vi "Read Resistance Setpoint.vi"   [LabVIEW 2023, in "Resistance Control.lvclass"]
uses:
  Resistance Control.lvclass
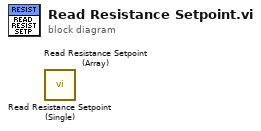
[diagram p0: block diagram]
diagram:
  n1 = call "Read Resistance Setpoint (Single).vi"() -> ()  [unwired: 8 in, 4 out]
  n2 = call "Read Resistance Setpoint (Array).vi"() -> ()  [unwired: 8 in, 4 out]
